vi "row modified.vi"(9 "OldVal":T1[](array[typedef]), 11 "NewVal":T1[](array[typedef])) -> (1 "Index":i32, 3 "Value Modified":T1={"App Name"="", "Build Type"=enum."Fix", "Current Version"="", "Next Version"="", "Check"=FALSE})   [LabVIEW 2021, in "App-Builder Library.lvlib" / "GUI Builder.lvclass"]
uses:
  GUI Builder.lvclass
  App descriptions.ctl
  Build Type.ctl
  Builder.lvclass
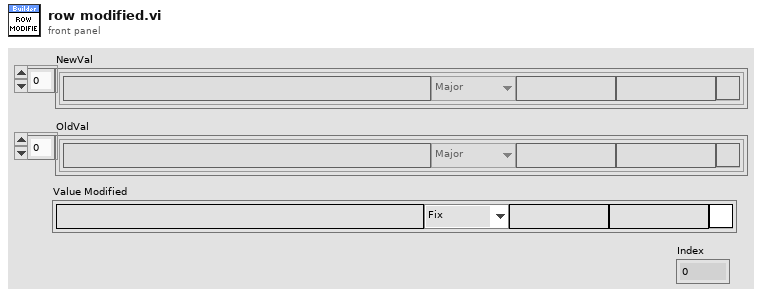
[diagram p1: front panel]
types:
  T1 = typedef "App-Builder Library.lvlib/Builder.lvclass/App descriptions.ctl" = cluster{"App Name":string, "Build Type":T2, "Current Version":string, "Next Version":string, "Check":bool}
  T2 = typedef "App-Builder Library.lvlib/Builder.lvclass/Build Type.ctl" = enum16{"Major", "Minor", "Fix", "Build"}
  T3 = cluster{"App Name":bool, "Build Type":bool, "Current Version":bool, "Next Version":bool, "Check":bool}
  T4 = cluster{"App Name":bool, "Build Type":bool, "Current Version":bool, "Next Version":bool, "Check":bool}[]
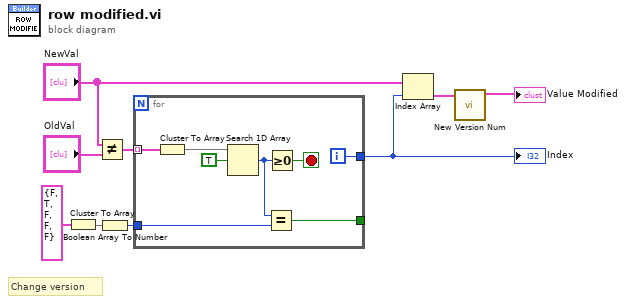
[diagram p0: block diagram]
diagram:
  # "Change version"
  n1 = Cluster To Array(cluster=T3 {"App Name"=FALSE, "Build Type"=TRUE, "Current Version"=FALSE, "Next Version"=FALSE, "Check"=FALSE} ("Applications")) -> (array=w4:bool[])
  n2 = Not Equal?(x="NewVal", y="OldVal") -> (x != y?=w9:T4)
  n3 = Boolean Array To Number(Boolean array=w4) -> (number=w3:u32)
  n4 = for {
    tunnel: w9 -> [w17] mode=indexing
    tunnel: [w13] -> w6
    tunnel: w3 -> [w11]
    tunnel: [w10] -> _
    i -> [w13]
    stop <- w14 stop-if-true
    n5 = Cluster To Array(cluster=w17) -> (array=w16:bool[])
    n6 = Search 1D Array(1D array=w16, element=TRUE ("App Name")) -> (index of element=w12:i32)  [unwired: 1 in]
    n7 = Equal?(x=w12, y=w11) -> (x = y?=w10:bool)
    n8 = Greater Or Equal To 0?(x=w12) -> (x >= 0?=w14:bool)
  }
  "Index" <- w6
  n9 = Index Array(array="NewVal", index=w6) -> (element=w2:T1)
  n10 = call "New Version Num.vi"("build modified"=w2) -> ("build modified out"=→"Value Modified":T1)  [unwired: 9 in, 1 out]
